vi "Filter_File_Type.vi"(8 "error in (no error)":errorcluster, 10 "file types":string[](array[string]), 11 "IB_Source_File in":refnum<class "IB_Source_File.lvclass">) -> (0 "error out":errorcluster, 2 "pass?":bool, 3 "filtered model":refnum<class "IB_Source.lvclass">)   [LabVIEW 2020, in "IB_Source_File.lvclass"]
uses:
  <vilib>/AppBuilder/IB_Classes/Source/File/IB_Source_File.lvclass
  <vilib>/AppBuilder/IB_Classes/Source/File/IB_Source_File.lvclass/IB_Source_File.ctl
  <vilib>/AppBuilder/IB_Classes/Source/IB_Source.lvclass
  e:/builds/penguin/labview/branches/2020/dev/dist/vi.lib/AppBuilder/IB_Classes/Source/IB_Source.lvclass
  e:/builds/penguin/labview/branches/2020/dev/dist/vi.lib/AppBuilder/IB_Classes/Source/File/IB_Source_File.lvclass
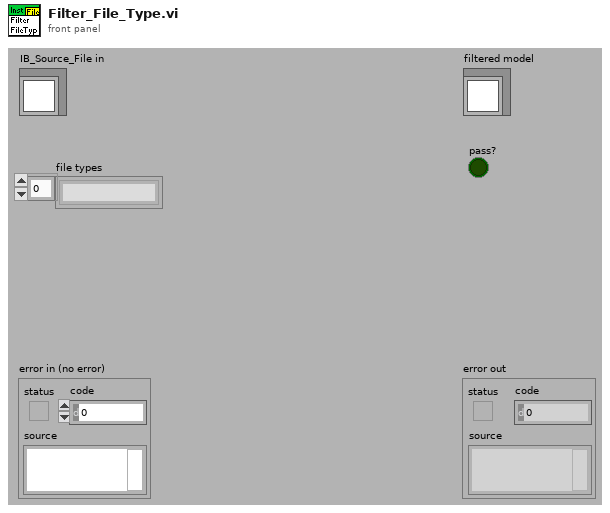
[diagram p1: front panel]
types:
  T1 = typedef "IB_Source.ctl" = cluster{"name":string, "sourceTag":string, "destTag":string, "path":path, "eng_installPath":string, "UI_inBuild?":bool, "str ref?":bool}
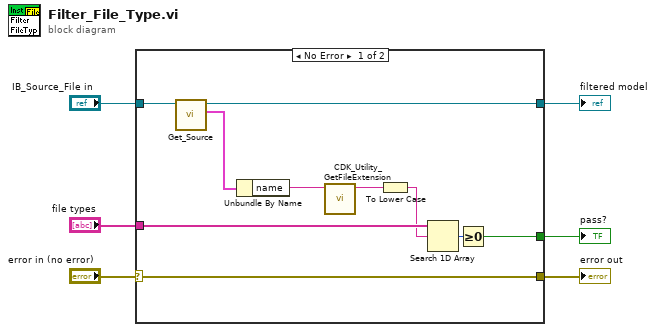
[diagram p0: block diagram]
diagram:
  n1 = case shown="No Error" "error in (no error)" {
    selector: "error in (no error)" -> [w9 w17]
    tunnel: "file types" -> [w16 _]
    tunnel: "IB_Source_File in" -> [w10 w18]
    tunnel: [w7 w18] -> w4
    tunnel: [w8 _] -> w3
    tunnel: [w9 w17] -> w1
    frame No Error {
      n2 = call <vilib>:"Get_Source.vi"("IB_Source in"=w10) -> ("data"=w11:T1, "IB_Source out"=w7:refnum<class "IB_Source_File.lvclass">)  [unwired: 1 in, 8 out]
      n3 = Unbundle By Name(w11) -> ("name"=w13:string)
      n4 = call <resource>:"CDK_Utility_GetFileExtension.vi"("filename"=w13) -> ("extension"=w12:string)  [unwired: 10 out]
      n5 = To Lower Case(string=w12) -> (all lower case string=w14:string)
      n6 = Search 1D Array(1D array=w16, element=w14) -> (index of element=w15:i32)  [unwired: 1 out]
      n7 = Greater Or Equal To 0?(x=w15) -> (x >= 0?=w8:bool)
    }
    frame Error {
    }
  }
  "error out" <- w1
  "filtered model" <- w4
  "pass?" <- w3
